vi "initialize debug mode.vi"(10 "User Event in":T1, 11 "editor node in":T2) -> (2 "User Event out":T1, 3 "editor node out":T2, 5 "engine":refnum<data-value>)   [LabVIEW 2014]
doc: "This VI creates dummy object references if the input references are invalid. Add test code here so that the editor can be run stand-alone."
uses:
  <vilib>/NI/Configuration Framework/Node/NodeRef.ctl
  <vilib>/NI/Configuration Framework/Node/NISE_CEF_Node.lvclass
  <vilib>/NI/Tag Bus Data Framework/Configuration Editor/Classes/Engine Parent/Engine Parent Editor Node.lvclass
  <vilib>/NI/Configuration Framework/Node/UserEventRef.ctl
  <vilib>/NI/Configuration Framework/Controls/EventCluster.ctl
  Simple Sequencer TBM editor node.lvclass
  module/configuration/Simple Sequencer TBM configuration.lvclass
  <vilib>/NI/Tag Bus Data Framework/Configuration Editor/Classes/Module editor node/Write Module Configuration.vi
  <vilib>/NI/Configuration Framework/NISE_CEF_TreeControl.lvlib
  <vilib>/NI/Tag Bus Data Framework/Configuration Editor/Classes/Module editor node/module editor node.lvclass
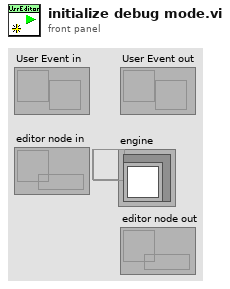
[diagram p1: front panel]
types:
  T1 = typedef "NISE_CEF_Node.lvclass/UserEventRef.ctl" = refnum<user-event>
  T2 = typedef "NISE_CEF_Node.lvclass/NodeRef.ctl" = refnum<data-value>
  T3 = typedef "NISE_CEF_TreeControl.lvlib/EventCluster.ctl" = cluster{"command":string, "data":string}
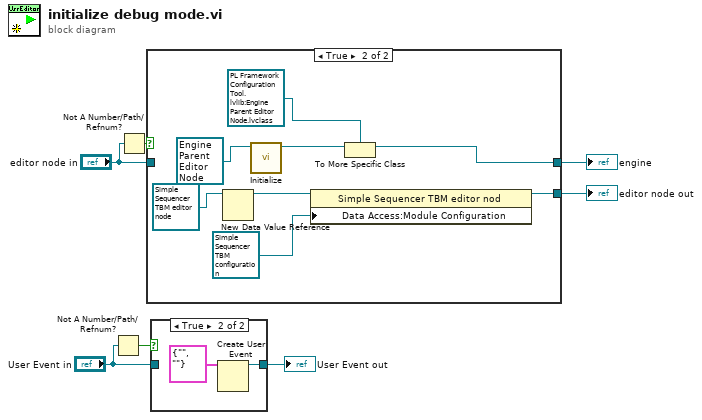
[diagram p0: block diagram]
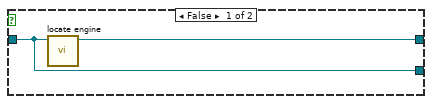
[diagram p3: hidden frame]
diagram:
  n1 = Not A Number/Path/Refnum?(number/path/refnum="User Event in") -> (NaN/Path/Refnum?=w3:bool)
  n2 = Not A Number/Path/Refnum?(number/path/refnum="editor node in") -> (NaN/Path/Refnum?=w4:bool)
  n3 = case shown="True" w4 {
    tunnel: "editor node in" -> [w8 _]
    tunnel: [w8 w17] -> w6
    tunnel: [w9 w15] -> w5
    frame False {
      n4 = call <vilib>:"locate engine.vi"("component"=w8) -> ("engine"=w9:refnum<data-value>)  [unwired: 9 in, 1 out]
    }
    frame True {
      n5 = New Data Value Reference(data value=refnum<class "Simple Sequencer TBM editor node.lvclass"> refnum ("tag bus configurable plugin editor node")) -> (data value reference=w13:refnum<data-value>)  [unwired: 1 in, 1 out]
      n6 = call-dynamic "Initialize.vi"("Engine in"=refnum<class "Engine Parent Editor Node.lvclass"> refnum ("PL Framework Configuration Tool.lvlib:Engine Parent Editor Node.lvclass")) -> ("data value reference"=w16:T2)  [unwired: 8 in, 2 out]
      n7 = property class="Simple Sequencer TBM editor nod"(reference=w13, "Data Access:Module Configuration"=refnum<class "Simple Sequencer TBM configuration.lvclass"> refnum ("user module configuration")) -> (reference out=w17:refnum<data-value>)  [unwired: 1 in, 1 out]
      n8 = To More Specific Class(target class=refnum<data-value> refnum ("data value reference"), reference=w16) -> (specific class reference=w15:refnum<data-value>)  [unwired: 1 in, 1 out]
    }
  }
  "editor node out" <- w6
  "engine" <- w5
  n9 = case shown="True" w3 {
    tunnel: "User Event in" -> [w18 _]
    tunnel: [w18 w19] -> w1
    frame False {
    }
    frame True {
      n10 = Create User Event(user event datatype=T3 {"command"="", "data"=""} ("event data")) -> (user event=w19:refnum<user-event>)  [unwired: 1 in, 1 out]
    }
  }
  "User Event out" <- w1
